vi "update position.vi"(8 "error in (no error)":errorcluster, 11 "focus in":refnum<class "focus.lvclass">) -> (0 "error out":errorcluster, 3 "focus out":refnum<class "focus.lvclass">)   [LabVIEW 2012, in "focus.lvclass"]
uses:
  focus.lvclass
  focus.lvclass/focus.ctl
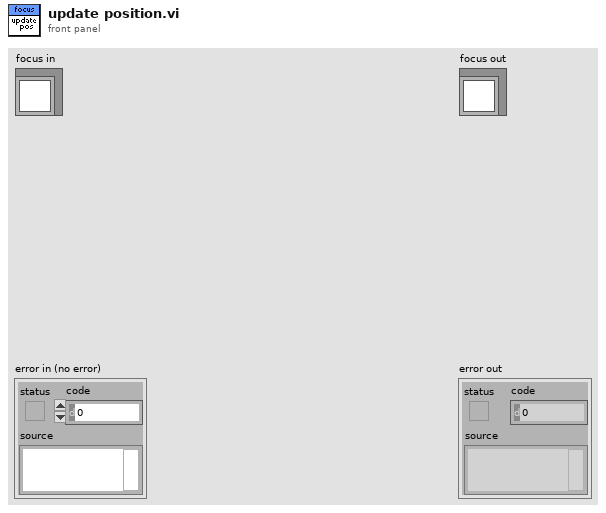
[diagram p1: front panel]
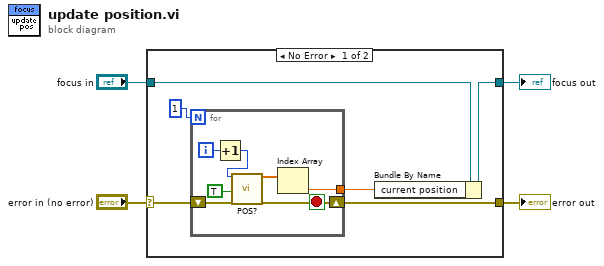
[diagram p0: block diagram]
diagram:
  n1 = case shown="No Error" "error in (no error)" {
    selector: "error in (no error)" -> [w9 w19]
    tunnel: [w5 w19] -> w3
    tunnel: [w6 w18] -> w1
    tunnel: "focus in" -> [w7 w18]
    frame No Error {
      n2 = for {
        N: 1 -> [_]
        shift-right: [w12] -> w5
        shift-left: w9 -> [w17]
        tunnel: [w11] -> w8
        i -> [w15]
        stop <- w12 stop-if-true
        n3 = Increment(x=w15) -> (x+1=w14:i32)
        n4 = call "POS?.vi"("System no."=w14, "All axes?"=TRUE, "error in"=w17) -> ("Position"=w13:dbl[], "error out"=w12:errorcluster)  [unwired: 15 in]
        n5 = Index Array(array=w13) -> (element=w11:dbl)  [unwired: 1 in]
      }
      n6 = Bundle By Name(cluster=w7, "current position"=w8) -> (w6:refnum<class "focus.lvclass">)
    }
    frame Error {
    }
  }
  "error out" <- w3
  "focus out" <- w1
